vi "Speed Limiter.vi"(1 "Max Allowed Speed [0, 1] (0)":dbl, 2 "Raw Speed In":dbl) -> (0 "Speed Limited Output":dbl)   [LabVIEW 2018]
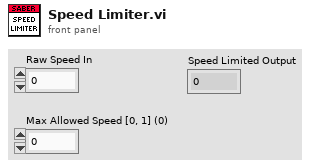
[diagram p1: front panel]
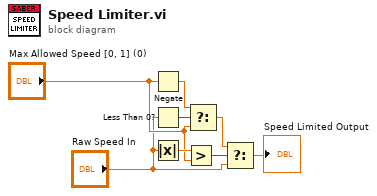
[diagram p0: block diagram]
diagram:
  n1 = Negate(x="Max Allowed Speed [0, 1] (0)") -> (-x=w4:dbl)
  n2 = Less Than 0?(x="Raw Speed In") -> (x < 0?=w5:bool)
  n3 = Absolute Value(x="Raw Speed In") -> (abs(x)=w8:dbl)
  n4 = Greater?(x=w8, y="Max Allowed Speed [0, 1] (0)") -> (0:w7:bool)
  n5 = Select(t=w4, s=w5, f="Max Allowed Speed [0, 1] (0)") -> (s? t:f=w2:dbl)
  n6 = Select(t=w2, s=w7, f="Raw Speed In") -> (s? t:f=→"Speed Limited Output":dbl)
